vi "Do.vi"(8 "error in (no error)":errorcluster, 10 "Actor in":refnum<class "Actor.lvclass">, 11 "SetGlobalThreshold":refnum<class "SetGlobalThresholdMsg.lvclass">) -> (0 "error out":errorcluster, 2 "Actor out":refnum<class "Actor.lvclass">)   [LabVIEW 2026, in "Lumberjack.lvlib" / "SetGlobalThresholdMsg.lvclass"]
doc: "<p>(<strong>Filename</strong>: <span class=\"dnl\">Actor Framework.lvlib:Message.lvclass:Do.vi</span>)</p>\n<p>Defines what a message does when it is received by an actor. Generally, a message instructs an actor to invoke one of its methods. By default, this method does nothing. A child class must override it to define behavior.</p>"
uses:
  SetGlobalThresholdMsg.lvclass
  <vilib>/ActorFramework/Actor/Actor.lvclass
  LogManager/LogManager.lvclass/LogManager.lvclass
  SetGlobalThresholdMsg.lvclass/SetGlobalThresholdMsg.ctl
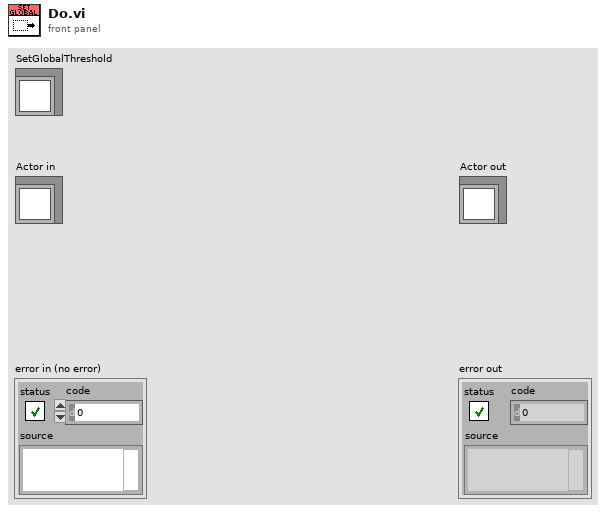
[diagram p1: front panel]
types:
  T1 = typedef "Lumberjack.lvlib/Severity.ctl" = enum16{"OFF", "FATAL", "ERROR", "WARN", "INFO", "DEBUG", "TRACE", "ALL"}
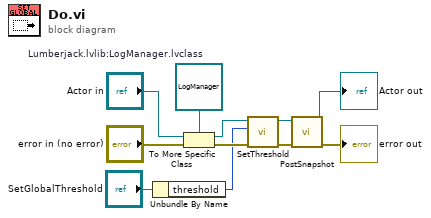
[diagram p0: block diagram]
diagram:
  w6 = refnum<class "LogManager.lvclass"> refnum  # Lumberjack.lvlib:LogManager.lvclass
  n1 = Unbundle By Name("SetGlobalThreshold") -> ("threshold"=w1:T1)
  n2 = To More Specific Class(target class=w6, reference="Actor in", error in="error in (no error)") -> (specific class reference=w4:refnum<class "LogManager.lvclass">, error out=w5:errorcluster)
  n3 = call "SetThreshold.vi"("error in (no error)"=w5, "Severity"=w1, "LogManager in"=w4) -> ("error out"=w2:errorcluster, "LogManager out"=w3:refnum<class "LogManager.lvclass">)  [unwired: 7 in]
  n4 = call "PostSnapshot.vi"("error in (no error)"=w2, "LogManager in"=w3) -> ("error out"=→"error out":errorcluster, "LogManager out"=→"Actor out":refnum<class "LogManager.lvclass">)  [unwired: 8 in]
